vi "DCC_Save2LVSET.vi"(6 "Overwrite Default File":bool, 7 "Array of Control Clusters":T1[](array[typedef]) {"Cooler Volt [V]" scale=0.0..5.0; "Cooler Current [A]" scale=0.0..2.0; "Connector 3"."Gain/HV [%]" scale=0.0..100.0; "Connector 1"."Gain/HV [%]" scale=0.0..100.0}, 8 "Error In":errorcluster) -> (0 "Error Out":errorcluster)   [LabVIEW 2019]
doc: "This function stores the DCC control cluster to a *.lvset file. The user can choose between two options. Write a new file or overwrite the default settings.\nThe default settings are normally the last stored settings of the \"SimpleMeasurement.vi\".\n\nMarch 2019\nFrank Quadt & Stefan Smietana\ninfo@becker-hickl.com"
uses:
  DCC_Controls/DCC_ControlCluster.ctl
  DCC_Controls/DCC_Connector1.ctl
  DCC_Controls/DCC_Connector2.ctl
panel:
  # "(c) 2018 Becker & Hickl GmbH\n     All Rights Reserved."
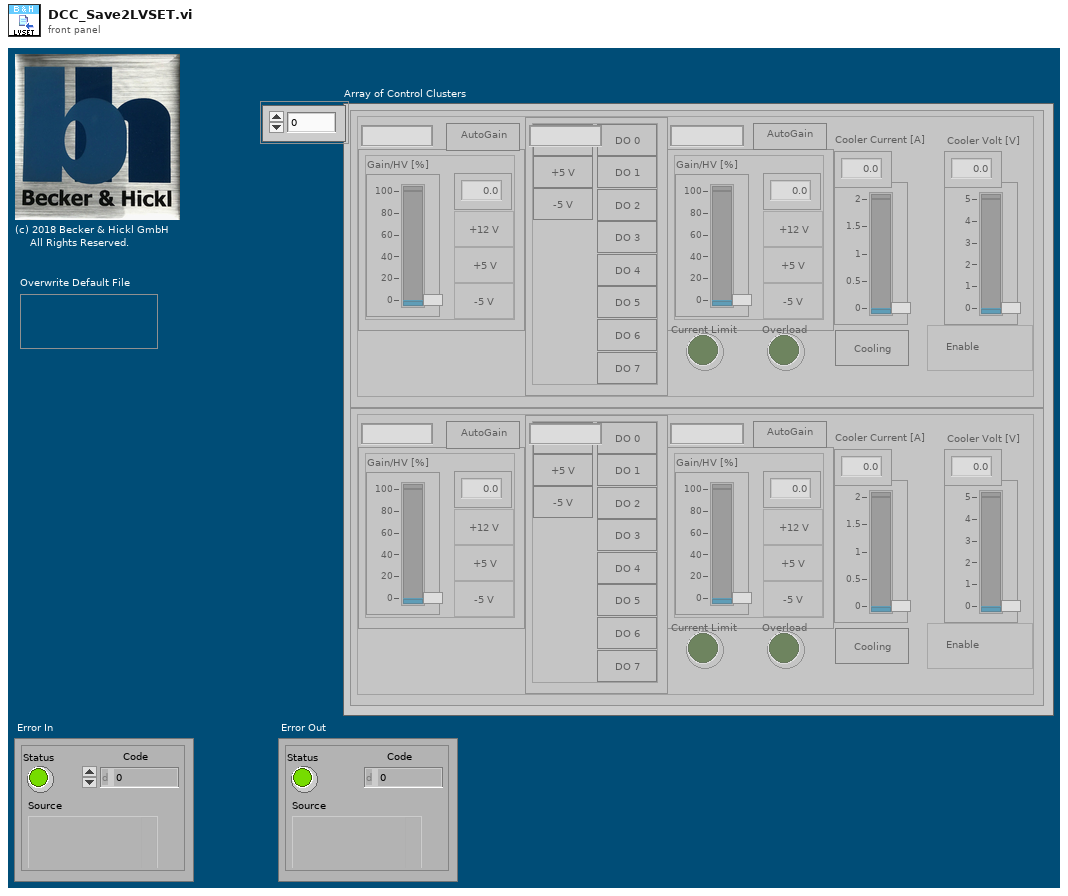
[diagram p1: front panel]
types:
  T1 = typedef "DCC_ControlCluster.ctl" = cluster{"Connector 1":T2, "Connector 2":T3, "Connector 3":T2, "Cooler Current [A]":dbl, "Cooler Volt [V]":dbl, "Cooling":bool, "Enable Outputs":bool, "AutoGain1":bool, "AutoGain3":bool, "Current Limit":bool, "Overload":bool, "LabelCon1":string, "LabelCon2":string, "LabelCon3":string}
  T2 = typedef "DCC_Connector1.ctl" = cluster{"Gain/HV [%]":dbl, "+12V":bool, "+5V":bool, "-5V":bool}
  T3 = typedef "DCC_Connector2.ctl" = cluster{"+12V":bool, "+5V":bool, "-5V":bool, "DO0":bool, "DO1":bool, "DO2":bool, "DO3":bool, "DO4":bool, "DO5":bool, "DO6":bool, "DO7":bool}
  T4 = enum16{"open", "replace", "create", "open or create", "replace or create", "replace or create with confirmation"}
  T5 = cluster{"[0]":u8, "[1]":u8, "[2]":u8, "[3]":u8, "[4]":u8, "[5]":u8, "[6]":u8, "[7]":u8, "[8]":u8, "[9]":u8, "[10]":u8, "[11]":u8, "[12]":u8, "[13]":u8, "[14]":u8, "[15]":u8}
  T6 = cluster{"Connector 1":T2, "Connector 2":T3, bool, bool, "Cooler Current [A]":dbl, "Cooler Volt [V]":dbl, bool, "Connector 3":T2, bool, cluster{"[0]":u8, "[1]":u8, "[2]":u8, "[3]":u8, "[4]":u8, "[5]":u8, "[6]":u8, "[7]":u8, "[8]":u8, "[9]":u8, "[10]":u8, "[11]":u8, "[12]":u8, "[13]":u8, "[14]":u8, "[15]":u8}, cluster{"[0]":u8, "[1]":u8, "[2]":u8, "[3]":u8, "[4]":u8, "[5]":u8, "[6]":u8, "[7]":u8, "[8]":u8, "[9]":u8, "[10]":u8, "[11]":u8, "[12]":u8, "[13]":u8, "[14]":u8, "[15]":u8}, cluster{"[0]":u8, "[1]":u8, "[2]":u8, "[3]":u8, "[4]":u8, "[5]":u8, "[6]":u8, "[7]":u8, "[8]":u8, "[9]":u8, "[10]":u8, "[11]":u8, "[12]":u8, "[13]":u8, "[14]":u8, "[15]":u8}}
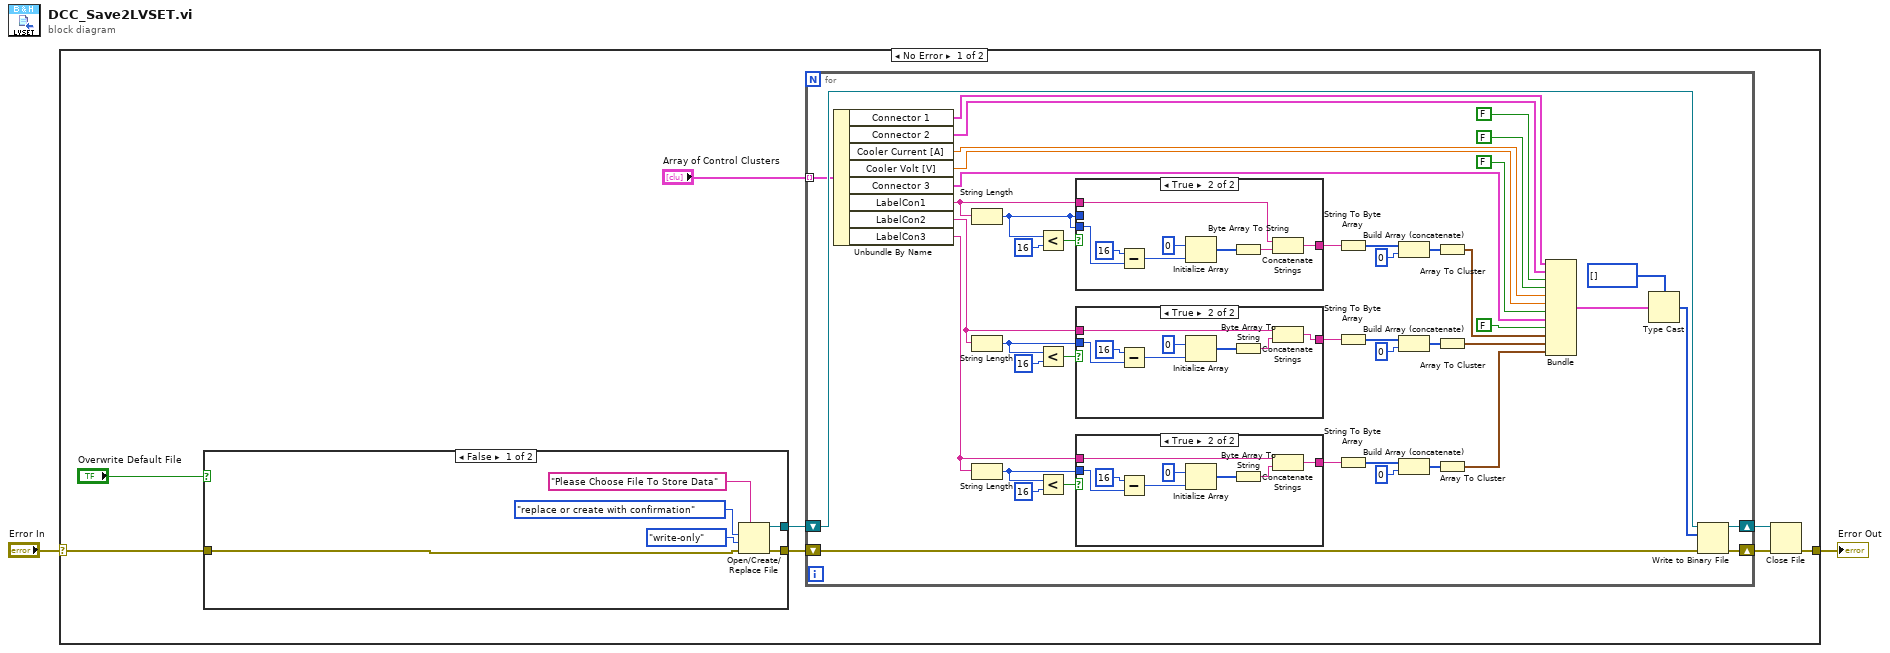
[diagram p0: block diagram]
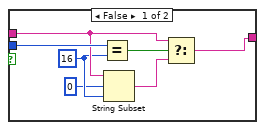
[diagram p2: hidden frame]
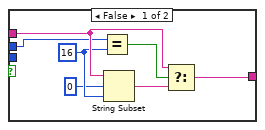
[diagram p3: hidden frame]
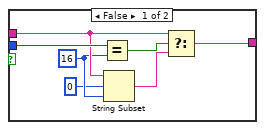
[diagram p4: hidden frame]
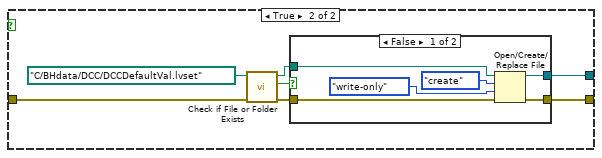
[diagram p5: hidden frame]
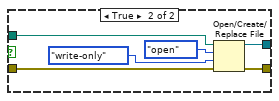
[diagram p6: hidden frame]
diagram:
  n1 = case shown="No Error" "Error In" {
    selector: "Error In" -> [w10 w125]
    tunnel: [w5 w125] -> w1
    frame No Error {
      n2 = case shown="False" "Overwrite Default File" {
        tunnel: w10 -> [w103 w108]
        tunnel: [w105 w107] -> w9
        tunnel: [w104 w106] -> w6
        frame False {
          n3 = Open/Create/Replace File(error in=w103, prompt="Please Choose File To Store Data", operation (0:open)=T4."replace or create with confirmation", access (0:read/write)=enum16{"read/write", "read-only", "write-only"}."write-only") -> (refnum out=w104:refnum<file>, error out=w105:errorcluster)  [unwired: 2 in, 1 out]
        }
        frame True {
          n4 = call <vilib>:"Check if File or Folder Exists.vi"("error in (no error)"=w108, "path"=path "C:/BHdata/DCC/DCCDefaultVal.lvset" ("file path (use dialog)")) -> ("error out"=w110:errorcluster, "file or folder exists?"=w112:bool, "dup path"=w111:path)  [unwired: 7 in]
          n5 = case shown="False" w112 {
            tunnel: w111 -> [w117 w124]
            tunnel: w110 -> [w118 w123]
            tunnel: [w114 w121] -> w107
            tunnel: [w113 w120] -> w106
            frame False {
              n6 = Open/Create/Replace File(file path (use dialog)=w117, error in=w118, operation (0:open)=T4."create", access (0:read/write)=enum16{"read/write", "read-only", "write-only"}."write-only") -> (refnum out=w113:refnum<file>, error out=w114:errorcluster)  [unwired: 2 in, 1 out]
            }
            frame True {
              n7 = Open/Create/Replace File(file path (use dialog)=w124, error in=w123, operation (0:open)=T4."open", access (0:read/write)=enum16{"read/write", "read-only", "write-only"}."write-only") -> (refnum out=w120:refnum<file>, error out=w121:errorcluster)  [unwired: 2 in, 1 out]
            }
          }
        }
      }
      n8 = for {
        shift-right: [w53] -> w8
        shift-left: w9 -> [w54]
        shift-right: [w52] -> w7
        shift-left: w6 -> [w51]
        tunnel: "Array of Control Clusters" -> [w26] mode=indexing
        n9 = Unbundle By Name(w26) -> ("Connector 1"=w50:T2, "Connector 2"=w49:T3, "Cooler Current [A]"=w48:dbl, "Cooler Volt [V]"=w47:dbl, "Connector 3"=w46:T2, "LabelCon1"=w12:string, "LabelCon2"=w11:string, "LabelCon3"=w19:string)
        n10 = String Length(string=w12) -> (length=w13:i32)
        n11 = String Length(string=w11) -> (length=w23:i32)
        n12 = String Length(string=w19) -> (length=w15:i32)
        n13 = Less?(x=w13, y=16) -> (x < y?=w18:bool)
        n14 = Less?(x=w23, y=16) -> (x < y?=w24:bool)
        n15 = Less?(x=w15, y=16) -> (x < y?=w14:bool)
        n16 = case shown="True" w18 {
          tunnel: w12 -> [w74 w84]
          tunnel: [w75 w78] -> w17
          tunnel: w13 -> [w70 _]
          tunnel: w13 -> [_ w77]
          frame False {
            w73 = 16
            n17 = Equal?(x=w70, y=w73) -> (x = y?=w76:bool)
            n18 = String Subset(string=w74, offset (0)=0, length (rest)=w73) -> (substring=w71:string)
            n19 = Select(t=w74, s=w76, f=w71) -> (s? t:f=w75:string)
          }
          frame True {
            n20 = Subtract(x=16, y=w77) -> (x-y=w82:i32)
            n21 = Initialize Array(u8 0, w82) -> (w80:u8[])
            n22 = Byte Array To String(unsigned byte array=w80) -> (string=w79:string)
            n23 = Concatenate Strings(w84, w79) -> (w78:string)
          }
        }
        n24 = case shown="True" w24 {
          tunnel: w11 -> [w88 w99]
          tunnel: w23 -> [w91 w97]
          tunnel: [w89 w92] -> w22
          frame False {
            w87 = 16
            n25 = Equal?(x=w91, y=w87) -> (x = y?=w90:bool)
            n26 = String Subset(string=w88, offset (0)=0, length (rest)=w87) -> (substring=w85:string)
            n27 = Select(t=w88, s=w90, f=w85) -> (s? t:f=w89:string)
          }
          frame True {
            n28 = Subtract(x=16, y=w97) -> (x-y=w96:i32)
            n29 = Initialize Array(u8 0, w96) -> (w94:u8[])
            n30 = Byte Array To String(unsigned byte array=w94) -> (string=w93:string)
            n31 = Concatenate Strings(w99, w93) -> (w92:string)
          }
        }
        n32 = case shown="True" w14 {
          tunnel: w19 -> [w58 w69]
          tunnel: w15 -> [w61 w67]
          tunnel: [w59 w62] -> w16
          frame False {
            w57 = 16
            n33 = Equal?(x=w61, y=w57) -> (x = y?=w60:bool)
            n34 = String Subset(string=w58, offset (0)=0, length (rest)=w57) -> (substring=w55:string)
            n35 = Select(t=w58, s=w60, f=w55) -> (s? t:f=w59:string)
          }
          frame True {
            n36 = Subtract(x=16, y=w67) -> (x-y=w66:i32)
            n37 = Initialize Array(u8 0, w66) -> (w64:u8[])
            n38 = Byte Array To String(unsigned byte array=w64) -> (string=w63:string)
            n39 = Concatenate Strings(w69, w63) -> (w62:string)
          }
        }
        n40 = String To Byte Array(string=w17) -> (unsigned byte array=w36:u8[])
        n41 = String To Byte Array(string=w22) -> (unsigned byte array=w38:u8[])
        n42 = String To Byte Array(string=w16) -> (unsigned byte array=w37:u8[])
        n43 = Build Array (concatenate)(w36, u8 0) -> (w39:u8[])
        n44 = Build Array (concatenate)(w38, u8 0) -> (w41:u8[])
        n45 = Build Array (concatenate)(w37, u8 0) -> (w40:u8[])
        n46 = Array To Cluster(array=w39) -> (cluster=w44:T5)
        n47 = Array To Cluster(array=w41) -> (cluster=w43:T5)
        n48 = Array To Cluster(array=w40) -> (cluster=w42:T5)
        n49 = Bundle("Connector 1"=w50, "Connector 2"=w49, FALSE, FALSE, "Cooler Current [A]"=w48, "Cooler Volt [V]"=w47, FALSE, "Connector 3"=w46, FALSE, w44, w43, w42) -> (w45:T6)  [unwired: 1 in]
        n50 = Type Cast(type=u8[] [], x=w45) -> (*(type *) &x=w27:u8[])
        n51 = Write to Binary File(file (use dialog)=w51, data=w27, error in=w54) -> (refnum out=w52:refnum<file>, error out=w53:errorcluster)  [unwired: 3 in, 1 out]
      }
      n52 = Close File(refnum=w7, error in=w8) -> (error out=w5:errorcluster)  [unwired: 1 out]
    }
    frame Error {
    }
  }
  "Error Out" <- w1
